vi "Density_Calc.vi"(8 "error in":errorcluster, 9 "R_air (ft*lbf)/(lbm*R)":dbl, 10 "T_in \n(Rankine: 70 Deg F + 460)":dbl, 11 "P_amb (psia)":dbl) -> (0 "error out":errorcluster, 3 "density":dbl)   [LabVIEW 2025]
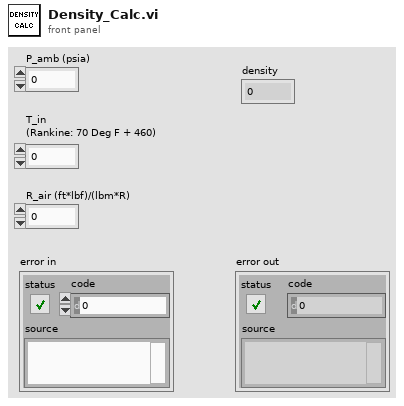
[diagram p1: front panel]
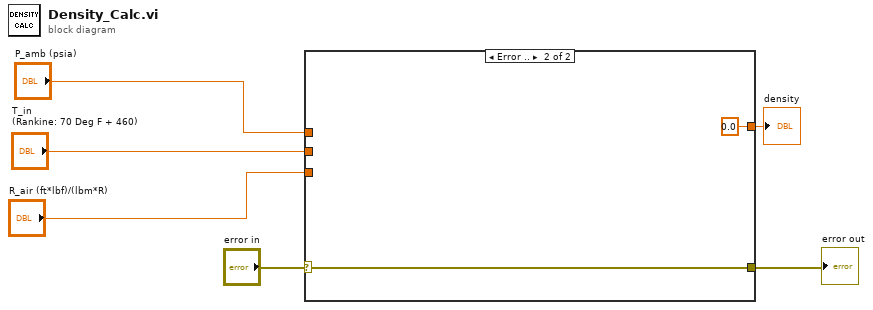
[diagram p0: block diagram]
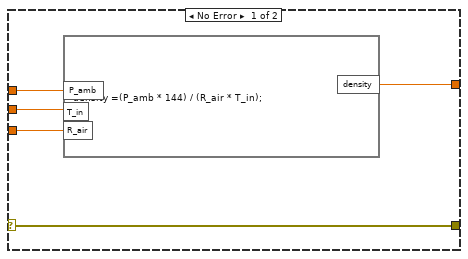
[diagram p2: hidden frame]
diagram:
  n1 = case shown="Error .." "error in" {
    selector: "error in" -> [w7 w13]
    tunnel: [w11 0.0 ("density")] -> w6
    tunnel: "P_amb (psia)" -> [w10 _]
    tunnel: "T_in \n(Rankine: 70 Deg F + 460)" -> [w9 _]
    tunnel: "R_air (ft*lbf)/(lbm*R)" -> [w8 _]
    tunnel: [w7 w13] -> w1
    frame No Error {
      n2 = formula code="density =(P_amb * 144) / (R_air * T_in);"("P_amb"=w10, "R_air"=w8, "T_in"=w9) -> ("density"=w11:dbl)
    }
    frame Error {
    }
  }
  "density" <- w6
  "error out" <- w1
